vi "NotARefNum.vi"(3 "reference in":refnum<class "Direction.lvclass">) -> (0 "not a refnum?":bool, 1 "reference out":refnum<class "Direction.lvclass">)   [LabVIEW 2013, in "Direction.lvclass"]
doc: "Checks if the specified object reference is valid."
uses:
  Direction.lvclass
  ObjectAttributesRef.ctl
  protected/ObjectAttributes.ctl
  Dec_class/Dec.lvclass
  Direction.lvclass/Direction.ctl
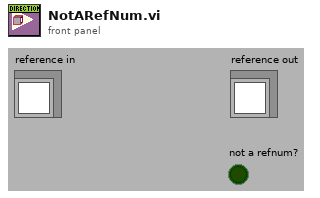
[diagram p1: front panel]
types:
  T1 = typedef "Direction.lvclass/ObjectAttributesRef.ctl" = refnum<data-value>
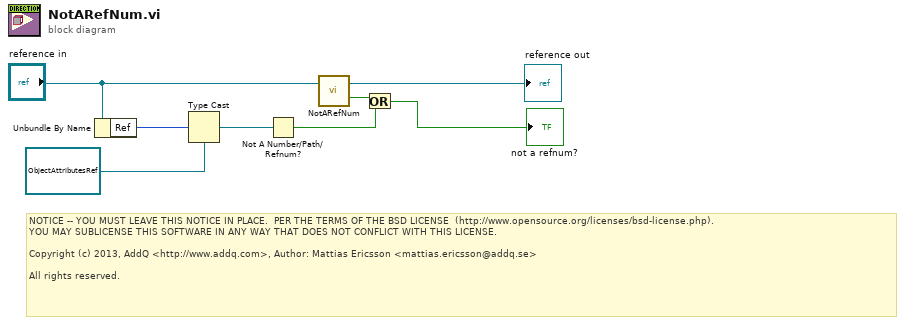
[diagram p0: block diagram]
diagram:
  # "NOTICE -- YOU MUST LEAVE THIS NOTICE IN PLACE.  PER THE TERMS OF THE BSD LICENSE  (http://www.opensource.org/licenses/bsd-license.php).\nYOU MAY SUBLICENSE THIS SOFTWARE IN ANY WAY THAT DOES NOT CONFLICT WITH THIS LICENSE.\n\nCopyright (c) 2013, AddQ <http://www.addq.com>, Author: Mattias Ericsson <mattias.ericsson@addq.se>\n\nAll rights reserved."
  n1 = Unbundle By Name("reference in") -> ("Ref"=w7:u32)
  n2 = Type Cast(type=T1 refnum ("attributes ref"), x=w7) -> (*(type *) &x=w6:T1)
  n3 = Not A Number/Path/Refnum?(number/path/refnum=w6) -> (NaN/Path/Refnum?=w2:bool)
  n4 = call-parent "NotARefNum.vi"("reference in"="reference in") -> ("not a refnum?"=w3:bool, "reference out"=→"reference out":refnum<class "Direction.lvclass">)  [unwired: 1 in]
  n5 = Or(x=w3, y=w2) -> (x .or. y?=→"not a refnum?":bool)
